vi "scan method parameters.Facade.vi"(0 "Data In":T5, 2 "Display State In":T3, 3 "Container State":T4) -> (6 "Data Out":T5, 7 "Display State Out":T3, 8 "Action":T2)   [LabVIEW 2014, in "PTScanner.lvlib" / "scan method parameters.xctl"]
uses:
  scan method parameters.xctl
  scan method parameters.Data.ctl
  <vilib>/_xctls/Container State.ctl
  scan method parameters.State.ctl
  <vilib>/_xctls/Action.ctl
  <vilib>/_xctls/XControlSupport.lvlib
  CSlibraries/UtilityLib/UtilityLib.lvlib
  _common/PTUtils/PTUtils.lvlib
panel:
  in  "Scrollbar":i32(c297)
  out "Indicator":T1
  in  "Control":T1
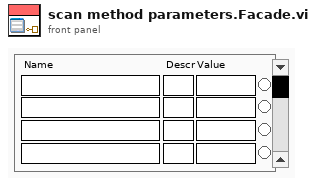
[diagram p1: front panel]
types:
  T1 = cluster{"Name 1":string, "Descr 1":string, "Value 1":string, "Value? 1":bool, "Name 2":string, "Descr 2":string, "Value 2":string, "Value? 2":bool, "Name 3":string, "Descr 3":string, "Value 3":string, "Value? 3":bool, "Name 4":string, "Descr 4":string, "Value 4":string, "Value? 4":bool}
  T2 = typedef "XControlSupport.lvlib/Action.ctl" = cluster{"Data Changed?":bool, "State Changed?":bool, "Action Name":string}
  T3 = typedef "PTScanner.lvlib/scan method parameters.xctl/scan method parameters.State.ctl" = cluster{"index":i32}
  T4 = typedef "XControlSupport.lvlib/Container State.ctl" = cluster{"Indicator?":bool, "Run Mode?":bool, " Refnum":refnum<vi>}
  T5 = typedef "PTScanner.lvlib/scan method parameters.xctl/scan method parameters.Data.ctl" = cluster{"Name":string, "Descr":string, "Value":string, "Value?":bool}[]
  T6 = enum8{"Enabled", "Disabled", "Disabled and Grayed Out"}
  T7 = cluster{"Name":string, "Descr":string, "Value":string, "Value?":bool}
  T8 = cluster{"Name":string, "Descr":string, "Value":string, "Value?":bool}[]
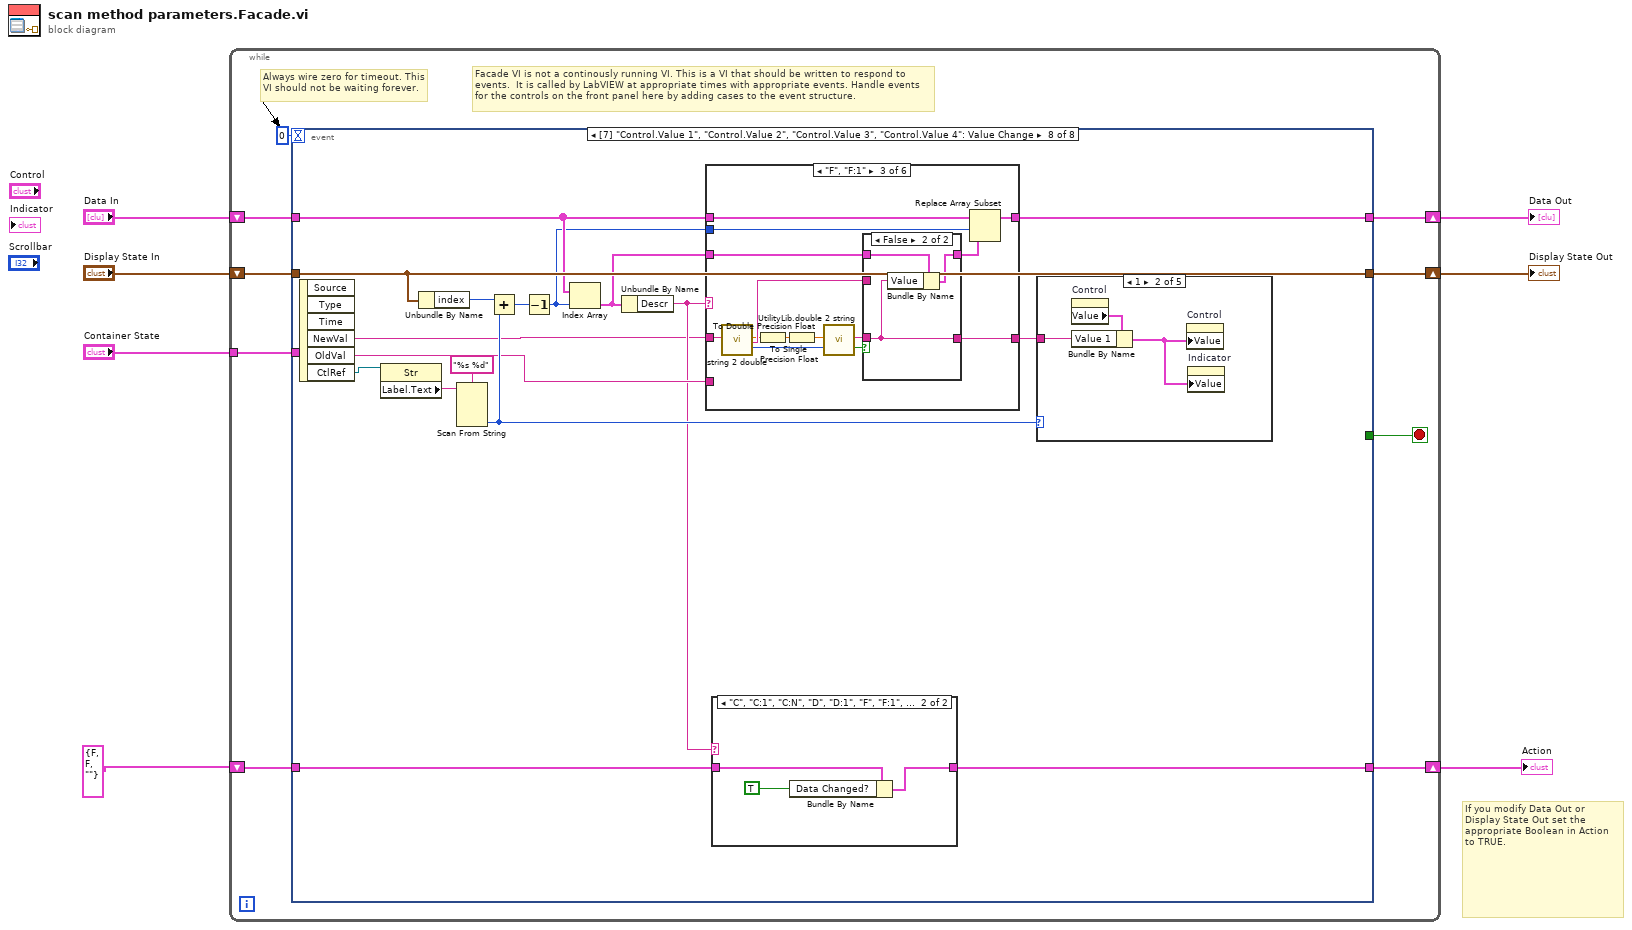
[diagram p0: block diagram]
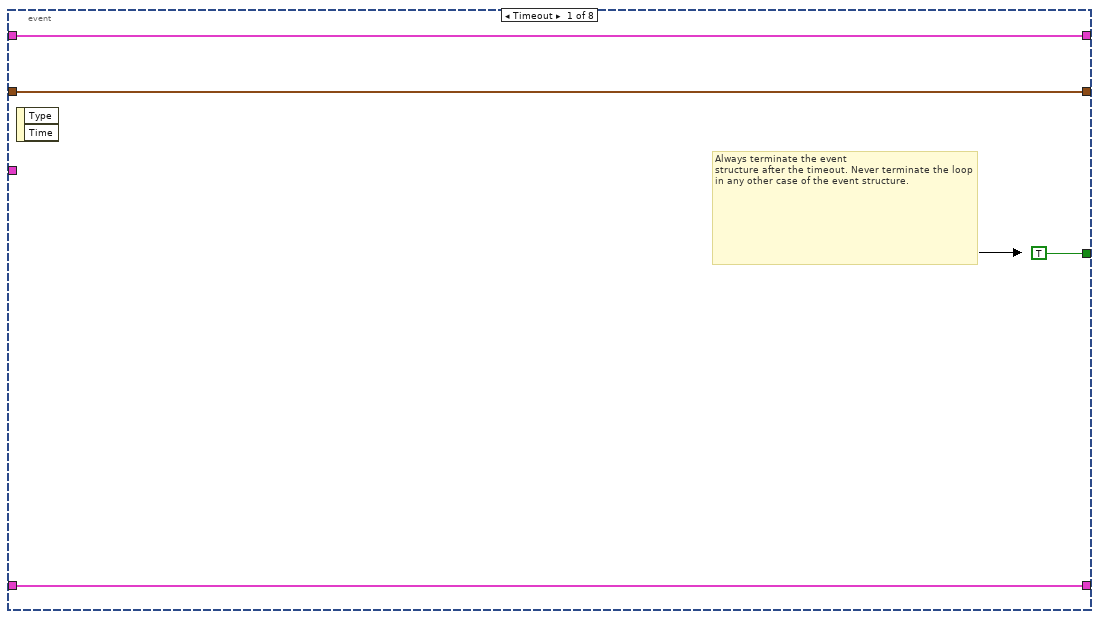
[diagram p2: hidden frame]
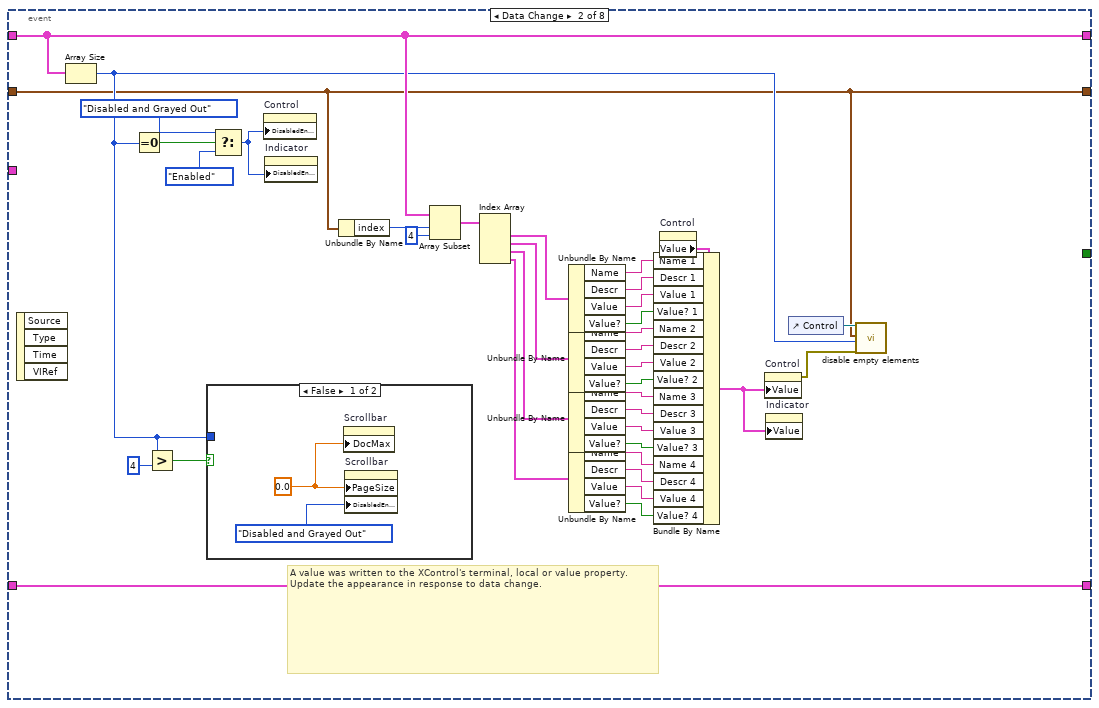
[diagram p3: hidden frame]
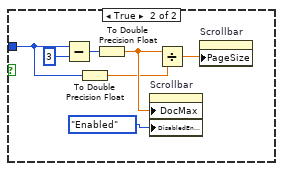
[diagram p4: hidden frame]
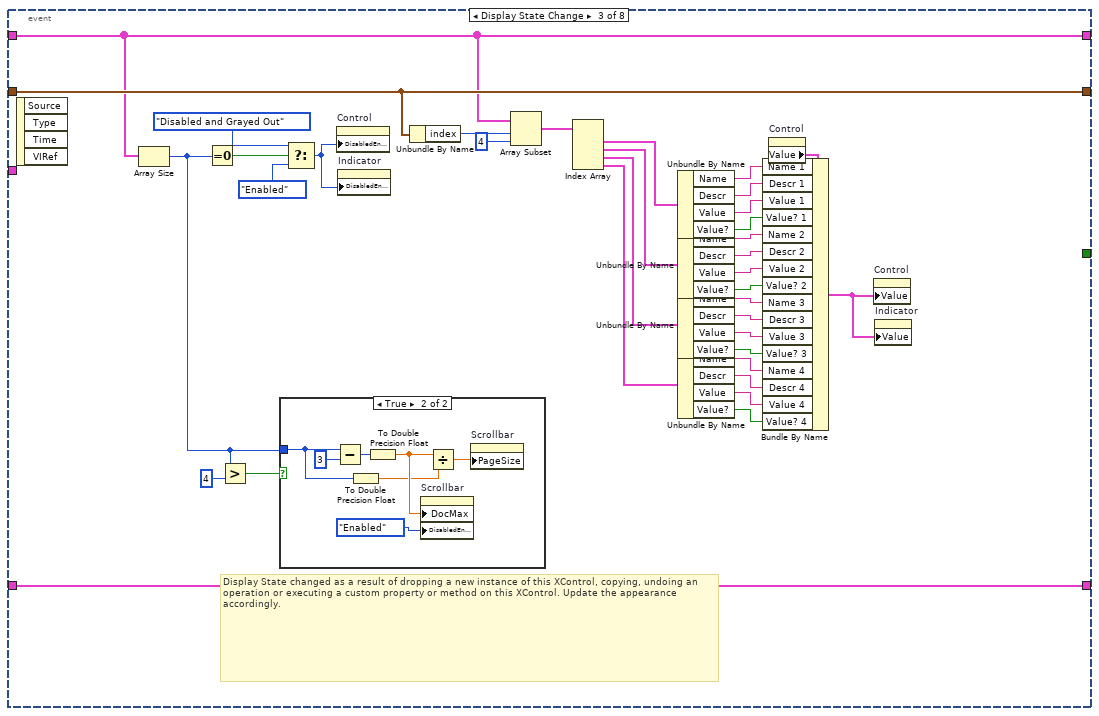
[diagram p5: hidden frame]
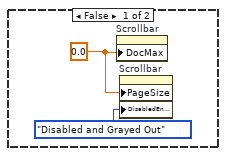
[diagram p6: hidden frame]
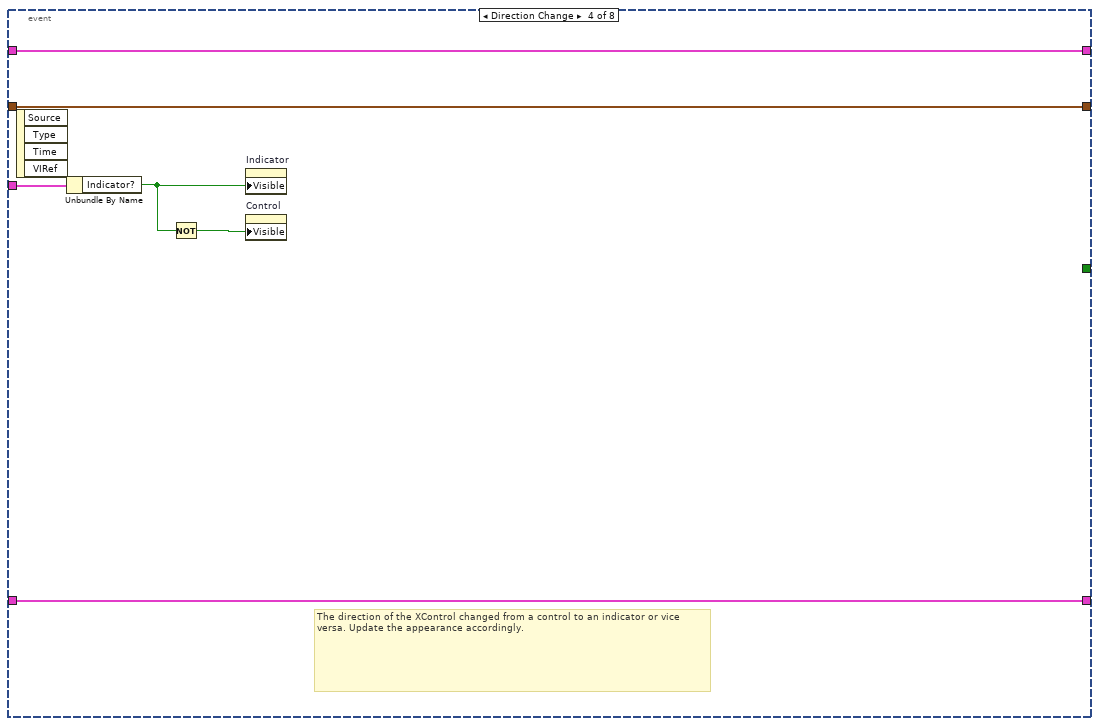
[diagram p7: hidden frame]
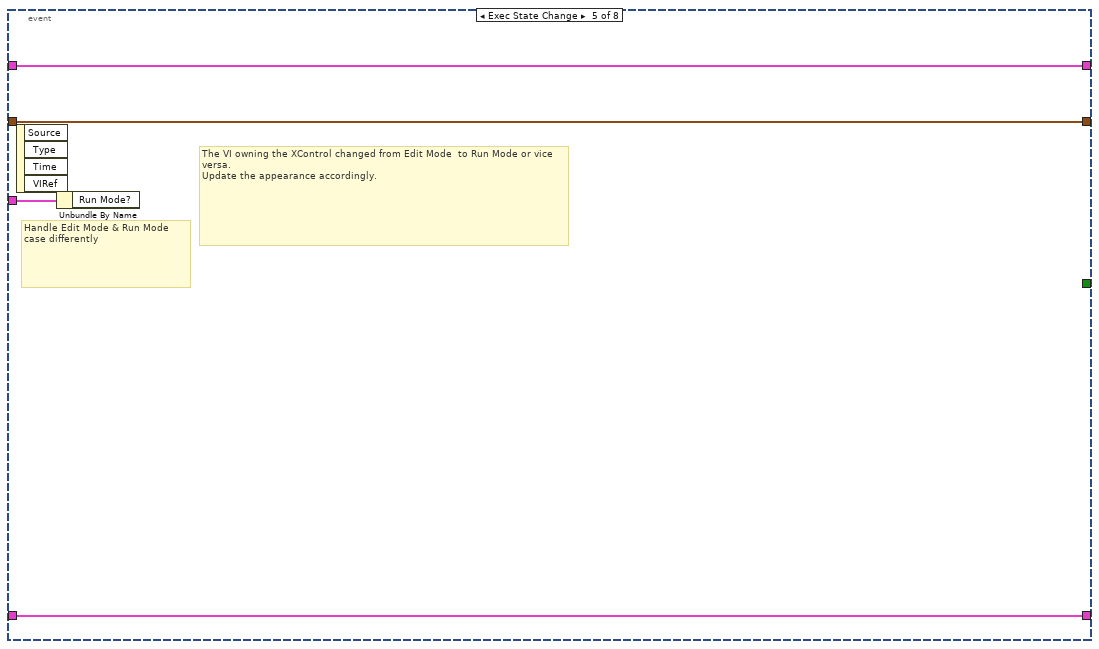
[diagram p8: hidden frame]
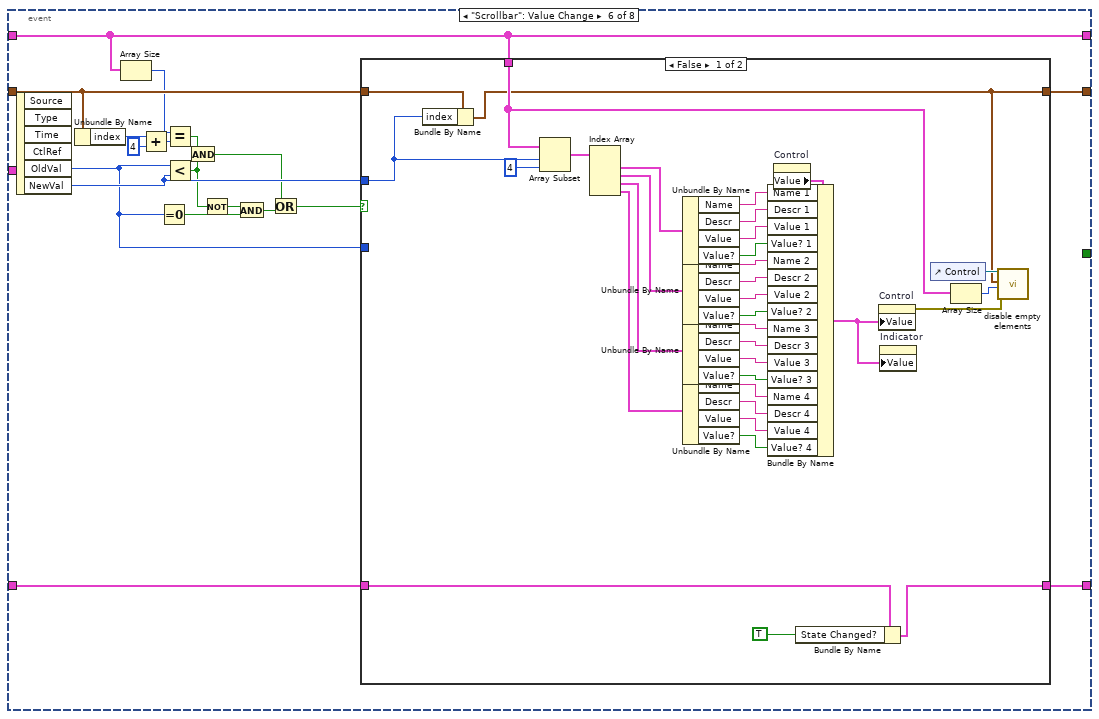
[diagram p9: hidden frame]
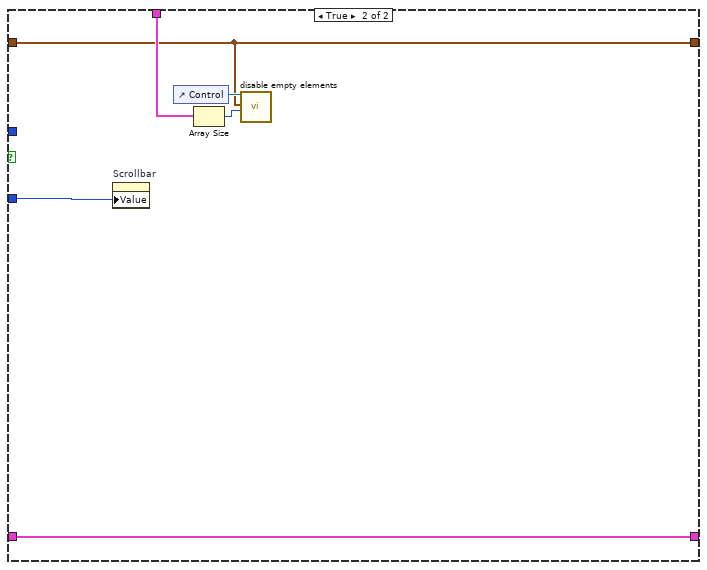
[diagram p10: hidden frame]
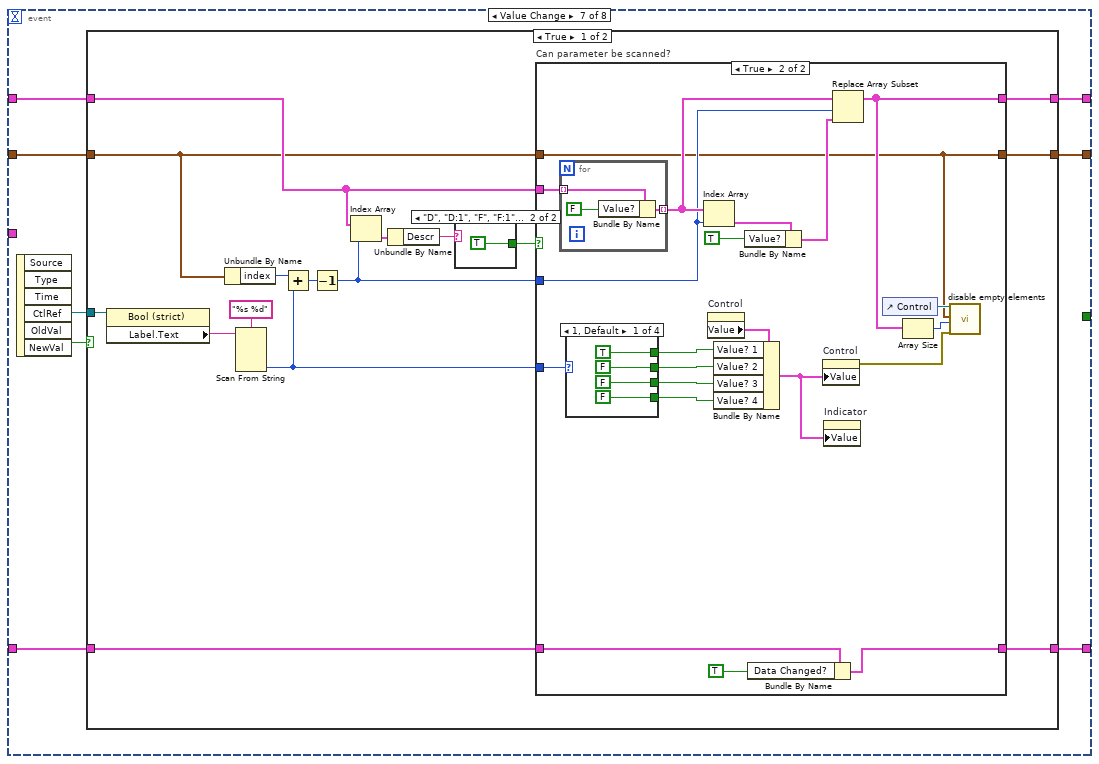
[diagram p11: hidden frame]
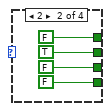
[diagram p13: hidden frame]
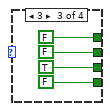
[diagram p14: hidden frame]
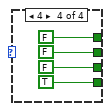
[diagram p15: hidden frame]
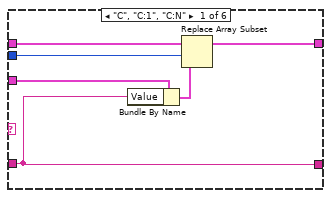
[diagram p19: hidden frame]
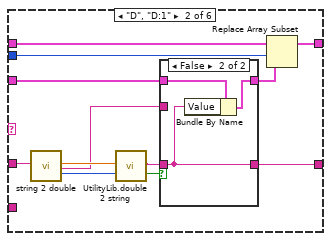
[diagram p20: hidden frame]
diagram:
  # "If you modify Data Out or\nDisplay State Out set the\nappropriate Boolean in Action\nto TRUE."
  n1 = while {
    shift-right: [w15] -> w4
    shift-left: "Display State In" -> [w16]
    tunnel: "Container State" -> [w12]
    shift-right: [w10] -> w7
    shift-left: "Data In" -> [w11]
    shift-right: [w8] -> w2
    shift-left: T2 {"Data Changed?"=FALSE, "State Changed?"=FALSE, "Action Name"=""} ("Action") -> [w9]
    stop <- w14 stop-if-true
    # "Facade VI is not a continously running VI. This is a VI that should be written to respond to events.  It is called by LabVIEW at appropriate times with appropriate events. Handle events for the controls on the front panel here by adding cases to the event structure."
    # "Always wire zero for timeout. This\nVI should not be waiting forever."
    n2 = event shown="[7] \"Control.Value 1\", \"Control.Value 2\", \"Control.Value 3\", \"Control.Value 4\": Value Change" {
      selector: _ -> [_ _ _ _ _ _ _ _]
      dyn-events: _ -> [_ _ _ _ _ _ _ _]
      timeout: 0 -> [_ _ _ _ _ _ _ _]
      tunnel: w16 -> [w18 w21 w100 w115 w119 w135 w183 w262]
      tunnel: [w18 w21 w100 w115 w119 w136 w182 w262] -> w15
      tunnel: [TRUE _ _ _ _ _ _ _] -> w14
      tunnel: w12 -> [_ _ _ w116 w120 _ _ _]
      tunnel: w11 -> [w17 w26 w67 w114 w118 w132 w184 w257]
      tunnel: [w17 w26 w67 w114 w118 w132 w185 w256] -> w10
      tunnel: [w19 w22 w101 w113 w117 w137 w181 w265] -> w8
      tunnel: w9 -> [w19 w22 w101 w113 w117 w138 w180 w266]
      event Timeout {
        # "Always terminate the event\nstructure after the timeout. Never terminate the loop in any other case of the event structure."
        n3 = event-data() -> ()  [unwired: 1 in, 2 out]
      }
      event Data Change {
        # "A value was written to the XControl's terminal, local or value property.\nUpdate the appearance in response to data change."
        n4 = event-data() -> ()  [unwired: 1 in, 4 out]
        n5 = Array Size(array=w26) -> (size(s)=w23:i32)
        n6 = Equal To 0?(x=w23) -> (x = 0?=w55:bool)
        n7 = Greater?(x=w23, y=4) -> (0:w52:bool)
        n8 = case shown="False" w52 {
          tunnel: w23 -> [_ w62]
          frame False {
            w58 = 0.0
            n9 = property on="Scrollbar" class="Scroll (strict)"("DocMax"=w58) -> ()  [unwired: 2 in, 2 out]
            n10 = property on="Scrollbar" class="Scroll (strict)"("PageSize"=w58, "DisabledEnum"=T6."Disabled and Grayed Out" ("Disabled")) -> ()  [unwired: 2 in, 2 out]
          }
          frame True {
            n11 = Subtract(x=w62, y=3) -> (x-y=w64:i32)
            n12 = To Double Precision Float(number=w62) -> (double precision float=w61:dbl)
            n13 = To Double Precision Float(number=w64) -> (double precision float=w63:dbl)
            n14 = property on="Scrollbar" class="Scroll (strict)"("DocMax"=w63, "DisabledEnum"=T6."Enabled" ("Disabled")) -> ()  [unwired: 2 in, 2 out]
            n15 = Divide(x=w63, y=w61) -> (x/y=w65:dbl)
            n16 = property on="Scrollbar" class="Scroll (strict)"("PageSize"=w65) -> ()  [unwired: 2 in, 2 out]
          }
        }
        n17 = Select(t=T6."Disabled and Grayed Out" ("Disabled"), s=w55, f=T6."Enabled" ("Disabled")) -> (s? t:f=w54:T6)
        n18 = property on="Control" class="Clust (strict)"("DisabledEnum"=w54) -> ()  [unwired: 2 in, 2 out]
        n19 = property on="Indicator" class="Clust (strict)"("DisabledEnum"=w54) -> ()  [unwired: 2 in, 2 out]
        n20 = Unbundle By Name(w21) -> ("index"=w51:i32)
        n21 = Array Subset(array=w26, index=w51, length=4) -> (w49:T5)
        n22 = Index Array(array=w49) -> (element #1=w47:T7, element #2=w46:T7, element #3=w45:T7, element #4=w44:T7)  [unwired: 4 in]
        n23 = Unbundle By Name(w47) -> ("Name"=w43:string, "Descr"=w42:string, "Value"=w41:string, "Value?"=w40:bool)
        n24 = Unbundle By Name(w46) -> ("Name"=w39:string, "Descr"=w38:string, "Value"=w37:string, "Value?"=w36:bool)
        n25 = Unbundle By Name(w45) -> ("Name"=w35:string, "Descr"=w34:string, "Value"=w33:string, "Value?"=w32:bool)
        n26 = Unbundle By Name(w44) -> ("Name"=w31:string, "Descr"=w30:string, "Value"=w29:string, "Value?"=w28:bool)
        n27 = property on="Control" class="Clust (strict)"() -> ("Value"=w48:T1)  [unwired: 2 in, 2 out]
        n28 = Bundle By Name(cluster=w48, "Name 1"=w43, "Descr 1"=w42, "Value 1"=w41, "Value? 1"=w40, "Name 2"=w39, "Descr 2"=w38, "Value 2"=w37, "Value? 2"=w36, "Name 3"=w35, "Descr 3"=w34, "Value 3"=w33, "Value? 3"=w32, "Name 4"=w31, "Descr 4"=w30, "Value 4"=w29, "Value? 4"=w28) -> (w27:T1)
        n29 = property on="Control" class="Clust (strict)"("Value"=w27) -> (error out=w24:errorcluster)  [unwired: 2 in, 1 out]
        n30 = property on="Indicator" class="Clust (strict)"("Value"=w27) -> ()  [unwired: 2 in, 2 out]
        n31 = control-ref of="Control"() -> (w25:refnum<vi>)
        n32 = call "disable empty elements.vi"("control ref"=w25, "State"=w21, "array size"=w23, "error in (no error)"=w24) -> ()  [unwired: 15 in, 1 out]
      }
      event Display State Change {
        # "Display State changed as a result of dropping a new instance of this XControl, copying, undoing an operation or executing a custom property or method on this XControl. Update the appearance accordingly."
        n33 = event-data() -> ()  [unwired: 1 in, 4 out]
        n34 = Array Size(array=w67) -> (size(s)=w68:i32)
        n35 = Equal To 0?(x=w68) -> (x = 0?=w72:bool)
        n36 = Greater?(x=w68, y=4) -> (0:w69:bool)
        n37 = case shown="True" w69 {
          tunnel: w68 -> [_ w106]
          frame False {
            w103 = 0.0
            n38 = property on="Scrollbar" class="Scroll (strict)"("DocMax"=w103) -> ()  [unwired: 2 in, 2 out]
            n39 = property on="Scrollbar" class="Scroll (strict)"("PageSize"=w103, "DisabledEnum"=T6."Disabled and Grayed Out" ("Disabled")) -> ()  [unwired: 2 in, 2 out]
          }
          frame True {
            n40 = Subtract(x=w106, y=3) -> (x-y=w108:i32)
            n41 = To Double Precision Float(number=w106) -> (double precision float=w105:dbl)
            n42 = To Double Precision Float(number=w108) -> (double precision float=w107:dbl)
            n43 = property on="Scrollbar" class="Scroll (strict)"("DocMax"=w107, "DisabledEnum"=T6."Enabled" ("Disabled")) -> ()  [unwired: 2 in, 2 out]
            n44 = Divide(x=w107, y=w105) -> (x/y=w109:dbl)
            n45 = property on="Scrollbar" class="Scroll (strict)"("PageSize"=w109) -> ()  [unwired: 2 in, 2 out]
          }
        }
        n46 = Select(t=T6."Disabled and Grayed Out" ("Disabled"), s=w72, f=T6."Enabled" ("Disabled")) -> (s? t:f=w71:T6)
        n47 = property on="Control" class="Clust (strict)"("DisabledEnum"=w71) -> ()  [unwired: 2 in, 2 out]
        n48 = property on="Indicator" class="Clust (strict)"("DisabledEnum"=w71) -> ()  [unwired: 2 in, 2 out]
        n49 = Unbundle By Name(w100) -> ("index"=w99:i32)
        n50 = Array Subset(array=w67, index=w99, length=4) -> (w97:T5)
        n51 = Index Array(array=w97) -> (element #1=w95:T7, element #2=w94:T7, element #3=w93:T7, element #4=w92:T7)  [unwired: 4 in]
        n52 = Unbundle By Name(w95) -> ("Name"=w91:string, "Descr"=w90:string, "Value"=w89:string, "Value?"=w88:bool)
        n53 = Unbundle By Name(w94) -> ("Name"=w87:string, "Descr"=w86:string, "Value"=w85:string, "Value?"=w84:bool)
        n54 = Unbundle By Name(w93) -> ("Name"=w83:string, "Descr"=w82:string, "Value"=w81:string, "Value?"=w80:bool)
        n55 = Unbundle By Name(w92) -> ("Name"=w79:string, "Descr"=w78:string, "Value"=w77:string, "Value?"=w76:bool)
        n56 = property on="Control" class="Clust (strict)"() -> ("Value"=w96:T1)  [unwired: 2 in, 2 out]
        n57 = Bundle By Name(cluster=w96, "Name 1"=w91, "Descr 1"=w90, "Value 1"=w89, "Value? 1"=w88, "Name 2"=w87, "Descr 2"=w86, "Value 2"=w85, "Value? 2"=w84, "Name 3"=w83, "Descr 3"=w82, "Value 3"=w81, "Value? 3"=w80, "Name 4"=w79, "Descr 4"=w78, "Value 4"=w77, "Value? 4"=w76) -> (w75:T1)
        n58 = property on="Control" class="Clust (strict)"("Value"=w75) -> ()  [unwired: 2 in, 2 out]
        n59 = property on="Indicator" class="Clust (strict)"("Value"=w75) -> ()  [unwired: 2 in, 2 out]
      }
      event Direction Change {
        # "The direction of the XControl changed from a control to an indicator or vice versa. Update the appearance accordingly."
        n60 = event-data() -> ()  [unwired: 1 in, 4 out]
        n61 = Unbundle By Name(w116) -> ("Indicator?"=w112:bool)
        n62 = Not(x=w112) -> (.not. x?=w111:bool)
        n63 = property on="Indicator" class="Clust (strict)"("Visible"=w112) -> ()  [unwired: 2 in, 2 out]
        n64 = property on="Control" class="Clust (strict)"("Visible"=w111) -> ()  [unwired: 2 in, 2 out]
      }
      event Exec State Change {
        # "The VI owning the XControl changed from Edit Mode  to Run Mode or vice versa.\nUpdate the appearance accordingly."
        # "Handle Edit Mode & Run Mode\ncase differently"
        n65 = event-data() -> ()  [unwired: 1 in, 4 out]
        n66 = Unbundle By Name(w120) -> ()  [unwired: 1 out]
      }
      event "Scrollbar": Value Change {
        n67 = event-data() -> ("OldVal"=w121:i32, "NewVal"=w129:i32)  [unwired: 1 in, 4 out]
        n68 = Unbundle By Name(w135) -> ("index"=w134:i32)
        n69 = Array Size(array=w132) -> (size(s)=w131:i32)
        n70 = Add(x=w134, y=4) -> (x+y=w130:i32)
        n71 = Equal To 0?(x=w121) -> (x = 0?=w125:bool)
        n72 = Equal?(x=w131, y=w130) -> (x = y?=w128:bool)
        n73 = Less?(x=w121, y=w129) -> (x < y?=w126:bool)
        n74 = And(x=w128, y=w126) -> (x .and. y?=w123:bool)
        n75 = Not(x=w126) -> (.not. x?=w127:bool)
        n76 = And(x=w127, y=w125) -> (x .and. y?=w124:bool)
        n77 = Or(x=w123, y=w124) -> (x .or. y?=w122:bool)
        n78 = case shown="False" w122 {
          tunnel: w138 -> [w172 w178]
          tunnel: [w171 w178] -> w137
          tunnel: [w139 w173] -> w136
          tunnel: w135 -> [w142 w173]
          tunnel: w132 -> [w140 w174]
          tunnel: w129 -> [w141 _]
          tunnel: w121 -> [_ w177]
          frame False {
            n79 = Bundle By Name(cluster=w142, "index"=w141) -> (w139:T3)
            n80 = Array Subset(array=w140, index=w141, length=4) -> (w168:T5)
            n81 = Index Array(array=w168) -> (element #1=w166:T7, element #2=w165:T7, element #3=w164:T7, element #4=w163:T7)  [unwired: 4 in]
            n82 = Unbundle By Name(w166) -> ("Name"=w162:string, "Descr"=w161:string, "Value"=w160:string, "Value?"=w159:bool)
            n83 = Unbundle By Name(w165) -> ("Name"=w158:string, "Descr"=w157:string, "Value"=w156:string, "Value?"=w155:bool)
            n84 = Unbundle By Name(w164) -> ("Name"=w154:string, "Descr"=w153:string, "Value"=w152:string, "Value?"=w151:bool)
            n85 = Unbundle By Name(w163) -> ("Name"=w150:string, "Descr"=w149:string, "Value"=w148:string, "Value?"=w147:bool)
            n86 = property on="Control" class="Clust (strict)"() -> ("Value"=w167:T1)  [unwired: 2 in, 2 out]
            n87 = Bundle By Name(cluster=w167, "Name 1"=w162, "Descr 1"=w161, "Value 1"=w160, "Value? 1"=w159, "Name 2"=w158, "Descr 2"=w157, "Value 2"=w156, "Value? 2"=w155, "Name 3"=w154, "Descr 3"=w153, "Value 3"=w152, "Value? 3"=w151, "Name 4"=w150, "Descr 4"=w149, "Value 4"=w148, "Value? 4"=w147) -> (w146:T1)
            n88 = Bundle By Name(cluster=w172, "State Changed?"=TRUE) -> (w171:T2)
            n89 = property on="Control" class="Clust (strict)"("Value"=w146) -> (error out=w143:errorcluster)  [unwired: 2 in, 1 out]
            n90 = property on="Indicator" class="Clust (strict)"("Value"=w146) -> ()  [unwired: 2 in, 2 out]
            n91 = control-ref of="Control"() -> (w145:refnum<vi>)
            n92 = Array Size(array=w140) -> (size(s)=w144:i32)
            n93 = call "disable empty elements.vi"("control ref"=w145, "State"=w139, "array size"=w144, "error in (no error)"=w143) -> ()  [unwired: 15 in, 1 out]
          }
          frame True {
            n94 = property on="Scrollbar" class="Scroll (strict)"("Value"=w177) -> ()  [unwired: 2 in, 2 out]
            n95 = control-ref of="Control"() -> (w176:refnum<vi>)
            n96 = Array Size(array=w174) -> (size(s)=w175:i32)
            n97 = call "disable empty elements.vi"("control ref"=w176, "State"=w173, "array size"=w175) -> ()  [unwired: 16 in, 1 out]
          }
        }
      }
      event "Control.Value? 1", "Control.Value? 2", "Control.Value? 3", "Control.Value? 4": Value Change {
        n98 = event-data() -> ("CtlRef"=w179:refnum<vi>, "NewVal"=w186:bool)  [unwired: 1 in, 4 out]
        n99 = case shown="True" w186 {
          tunnel: w179 -> [w202 _]
          tunnel: [w199 w248] -> w185
          tunnel: w184 -> [w194 w248]
          tunnel: w183 -> [w188 w249]
          tunnel: [w187 w249] -> w182
          tunnel: [w189 w247] -> w181
          tunnel: w180 -> [w190 w247]
          frame True {
            n100 = property class="Bool (strict)"(reference=w202) -> ("Label.Text"=w201:string)  [unwired: 1 in, 2 out]
            n101 = Unbundle By Name(w188) -> ("index"=w197:i32)
            n102 = Scan From String(format string="%s %d", input string=w201) -> (output 2=w198:i32)  [unwired: 5 in, 3 out]
            n103 = Add(x=w197, y=w198) -> (x+y=w196:i32)
            n104 = Decrement(x=w196) -> (x-1=w195:i32)
            n105 = Index Array(array=w194, index=w195) -> (element=w193:T7)
            n106 = Unbundle By Name(w193) -> ("Descr"=w192:string)
            n107 = case shown="\"D\", \"D:1\", \"F\", \"F:1\", \"I\", \"I:1\", \"L\", \"L:1\"" w192 {
              tunnel: [_ TRUE] -> w191
              frame "", Default {
              }
              frame "D", "D:1", "F", "F:1", "I", "I:1", "L", "L:1" {
              }
            }
            n108 = case "Can parameter be scanned?" shown="True" w191 {
              tunnel: [w205 w217] -> w199
              tunnel: w198 -> [_ w216]
              tunnel: w195 -> [_ w211]
              tunnel: w194 -> [w205 w210]
              tunnel: w190 -> [w204 w208]
              tunnel: [w204 w207] -> w189
              tunnel: w188 -> [w203 w206]
              tunnel: [w203 w206] -> w187
              frame False {
              }
              frame True {
                n109 = for {
                  tunnel: w210 -> [w229] mode=indexing
                  tunnel: [w227] -> w215 mode=indexing
                  n110 = Bundle By Name(cluster=w229, "Value?"=FALSE) -> (w227:T7)
                }
                n111 = case shown="1, Default" w216 {
                  tunnel: [TRUE FALSE FALSE FALSE] -> w224
                  tunnel: [FALSE TRUE FALSE FALSE] -> w223
                  tunnel: [FALSE FALSE TRUE FALSE] -> w222
                  tunnel: [FALSE FALSE FALSE TRUE] -> w221
                  frame 1, Default {
                  }
                  frame 2 {
                  }
                  frame 3 {
                  }
                  frame 4 {
                  }
                }
                n112 = Index Array(array=w215, index=w211) -> (element=w214:T7)
                n113 = property on="Control" class="Clust (strict)"() -> ("Value"=w226:T1)  [unwired: 2 in, 2 out]
                n114 = Bundle By Name(cluster=w226, "Value? 1"=w224, "Value? 2"=w223, "Value? 3"=w222, "Value? 4"=w221) -> (w225:T1)
                n115 = Bundle By Name(cluster=w214, "Value?"=TRUE) -> (w212:T7)
                n116 = Bundle By Name(cluster=w208, "Data Changed?"=TRUE) -> (w207:T2)
                n117 = property on="Control" class="Clust (strict)"("Value"=w225) -> (error out=w218:errorcluster)  [unwired: 2 in, 1 out]
                n118 = property on="Indicator" class="Clust (strict)"("Value"=w225) -> ()  [unwired: 2 in, 2 out]
                n119 = Replace Array Subset(array=w215, new element=w212, index=w211) -> (w217:T8)
                n120 = control-ref of="Control"() -> (w220:refnum<vi>)
                n121 = Array Size(array=w217) -> (size(s)=w219:i32)
                n122 = call "disable empty elements.vi"("control ref"=w220, "State"=w206, "array size"=w219, "error in (no error)"=w218) -> ()  [unwired: 15 in, 1 out]
              }
            }
          }
          frame False {
          }
        }
      }
      event "Control.Value 1", "Control.Value 2", "Control.Value 3", "Control.Value 4": Value Change {
        n123 = event-data() -> ("NewVal"=w250:string, "OldVal"=w253:string, "CtlRef"=w258:refnum<vi>)  [unwired: 1 in, 3 out]
        n124 = property class="Str"(reference=w258) -> ("Label.Text"=w264:string)  [unwired: 1 in, 2 out]
        n125 = Unbundle By Name(w262) -> ("index"=w261:i32)
        n126 = Scan From String(format string="%s %d", input string=w264) -> (output 2=w259:i32)  [unwired: 5 in, 3 out]
        n127 = Add(x=w261, y=w259) -> (x+y=w260:i32)
        n128 = Decrement(x=w260) -> (x-1=w254:i32)
        n129 = Index Array(array=w257, index=w254) -> (element=w255:T7)
        n130 = Unbundle By Name(w255) -> ("Descr"=w251:string)
        n131 = case shown="\"F\", \"F:1\"" w251 {
          tunnel: w257 -> [w275 w288 w308 w318 w329 w335]
          tunnel: [w276 w287 w307 w319 w328 w335] -> w256
          tunnel: w250 -> [w271 w283 w303 w324 w333 _]
          tunnel: [w271 w278 w299 w316 w326 w334] -> w252
          tunnel: w255 -> [w273 w286 w306 w317 w327 _]
          tunnel: w254 -> [w274 w284 w304 w315 w325 _]
          tunnel: w253 -> [_ _ _ _ _ w334]
          frame "C", "C:1", "C:N" {
            n132 = Bundle By Name(cluster=w273, "Value"=w271) -> (w272:T7)
            n133 = Replace Array Subset(array=w275, new element=w272, index=w274) -> (w276:T5)
          }
          frame "D", "D:1" {
            n134 = call "string 2 double.vi"("string"=w283) -> ("number"=w282:dbl, "scanned string"=w279:string, "length"=w281:u8)  [unwired: 15 in, 1 out]
            n135 = call "UtilityLib.double 2 string.vi"("Numeric"=w282, "length"=w281) -> ("String"=w277:string, "loss free"=w280:bool)  [unwired: 16 in]
            n136 = case shown="False" w280 {
              tunnel: w286 -> [w291 w294]
              tunnel: [w290 w293] -> w285
              tunnel: w279 -> [w289 _]
              tunnel: [w289 w292] -> w278
              tunnel: w277 -> [_ w292]
              frame True {
                n137 = Bundle By Name(cluster=w291, "Value"=w289) -> (w290:T7)
              }
              frame False {
                n138 = Bundle By Name(cluster=w294, "Value"=w292) -> (w293:T7)
              }
            }
            n139 = Replace Array Subset(array=w288, new element=w285, index=w284) -> (w287:T5)
          }
          frame "F", "F:1" {
            n140 = call "string 2 double.vi"("string"=w303) -> ("number"=w298:dbl, "scanned string"=w300:string, "length"=w302:u8)  [unwired: 15 in, 1 out]
            n141 = To Single Precision Float(number=w298) -> (single precision float=w297:sgl)
            n142 = To Double Precision Float(number=w297) -> (double precision float=w296:dbl)
            n143 = call "UtilityLib.double 2 string.vi"("Numeric"=w296, "length"=w302) -> ("String"=w295:string, "loss free"=w301:bool)  [unwired: 16 in]
            n144 = case shown="False" w301 {
              tunnel: w306 -> [w311 w314]
              tunnel: [w310 w313] -> w305
              tunnel: w300 -> [w309 _]
              tunnel: [w309 w312] -> w299
              tunnel: w295 -> [_ w312]
              frame True {
                n145 = Bundle By Name(cluster=w311, "Value"=w309) -> (w310:T7)
              }
              frame False {
                n146 = Bundle By Name(cluster=w314, "Value"=w312) -> (w313:T7)
              }
            }
            n147 = Replace Array Subset(array=w308, new element=w305, index=w304) -> (w307:T5)
          }
          frame "S", "S:1" {
            n148 = Decimal String To Number(string=w324, default (0L)=i16 0) -> (number=w322:i16)  [unwired: 1 in, 1 out]
            n149 = Format Into String(format string="%d", w322) -> (resulting string=w316:string)  [unwired: 2 in, 1 out]
            n150 = Bundle By Name(cluster=w317, "Value"=w316) -> (w320:T7)
            n151 = Replace Array Subset(array=w318, new element=w320, index=w315) -> (w319:T5)
          }
          frame "I", "I:1", "L", "L:1" {
            n152 = Decimal String To Number(string=w333) -> (number=w332:i32)  [unwired: 2 in, 1 out]
            n153 = Format Into String(format string="%d", w332) -> (resulting string=w326:string)  [unwired: 2 in, 1 out]
            n154 = Bundle By Name(cluster=w327, "Value"=w326) -> (w330:T7)
            n155 = Replace Array Subset(array=w329, new element=w330, index=w325) -> (w328:T5)
          }
          frame Default {
          }
        }
        n156 = case shown="\"C\", \"C:1\", \"C:N\", \"D\", \"D:1\", \"F\", \"F:1\", \"I\", \"I:1\", \"L\", \"L:1\", \"S\", \"S:1\"" w251 {
          tunnel: w266 -> [w267 w270]
          tunnel: [w267 w269] -> w265
          frame "", Default {
          }
          frame "C", "C:1", "C:N", "D", "D:1", "F", "F:1", "I", "I:1", "L", "L:1", "S", "S:1" {
            n157 = Bundle By Name(cluster=w270, "Data Changed?"=TRUE) -> (w269:T2)
          }
        }
        n158 = case shown="1" w259 {
          tunnel: w252 -> [_ w336 w339 w342 w345]
          frame 0, Default {
          }
          frame 1 {
            n159 = property on="Control" class="Clust (strict)"() -> ("Value"=w338:T1)  [unwired: 2 in, 2 out]
            n160 = Bundle By Name(cluster=w338, "Value 1"=w336) -> (w337:T1)
            n161 = property on="Control" class="Clust (strict)"("Value"=w337) -> ()  [unwired: 2 in, 2 out]
            n162 = property on="Indicator" class="Clust (strict)"("Value"=w337) -> ()  [unwired: 2 in, 2 out]
          }
          frame 2 {
            n163 = property on="Control" class="Clust (strict)"() -> ("Value"=w341:T1)  [unwired: 2 in, 2 out]
            n164 = Bundle By Name(cluster=w341, "Value 2"=w339) -> (w340:T1)
            n165 = property on="Control" class="Clust (strict)"("Value"=w340) -> ()  [unwired: 2 in, 2 out]
            n166 = property on="Indicator" class="Clust (strict)"("Value"=w340) -> ()  [unwired: 2 in, 2 out]
          }
          frame 3 {
            n167 = property on="Control" class="Clust (strict)"() -> ("Value"=w344:T1)  [unwired: 2 in, 2 out]
            n168 = Bundle By Name(cluster=w344, "Value 3"=w342) -> (w343:T1)
            n169 = property on="Control" class="Clust (strict)"("Value"=w343) -> ()  [unwired: 2 in, 2 out]
            n170 = property on="Indicator" class="Clust (strict)"("Value"=w343) -> ()  [unwired: 2 in, 2 out]
          }
          frame 4 {
            n171 = property on="Control" class="Clust (strict)"() -> ("Value"=w347:T1)  [unwired: 2 in, 2 out]
            n172 = Bundle By Name(cluster=w347, "Value 4"=w345) -> (w346:T1)
            n173 = property on="Control" class="Clust (strict)"("Value"=w346) -> ()  [unwired: 2 in, 2 out]
            n174 = property on="Indicator" class="Clust (strict)"("Value"=w346) -> ()  [unwired: 2 in, 2 out]
          }
        }
      }
    }
  }
  "Display State Out" <- w4
  "Data Out" <- w7
  "Action" <- w2
